vi "array percentage.vi"(8 "path":path=path "D:/Data/20200212_test", 9 "Array":dbl[](array[numeric]), 10 "Judgement value":dbl format="%#_13g") -> ()   [LabVIEW 2018]
uses:
  <vilib>/Utility/file.llb/Read From Spreadsheet File (DBL).vi
panel:
  out "read in array":dbl[](array[numeric])
  # "output the index and element of an array that smaller or equal that judgement value"
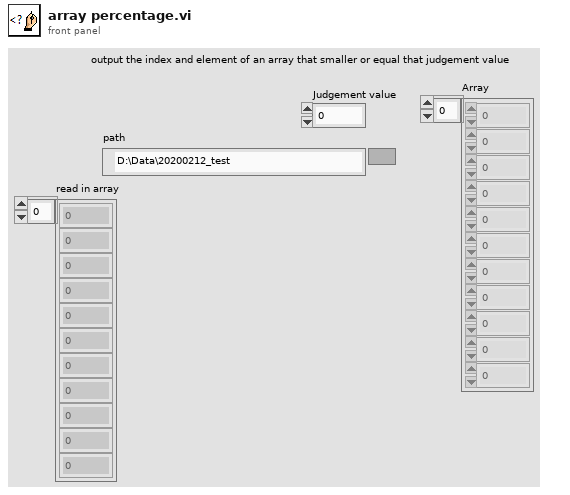
[diagram p1: front panel]
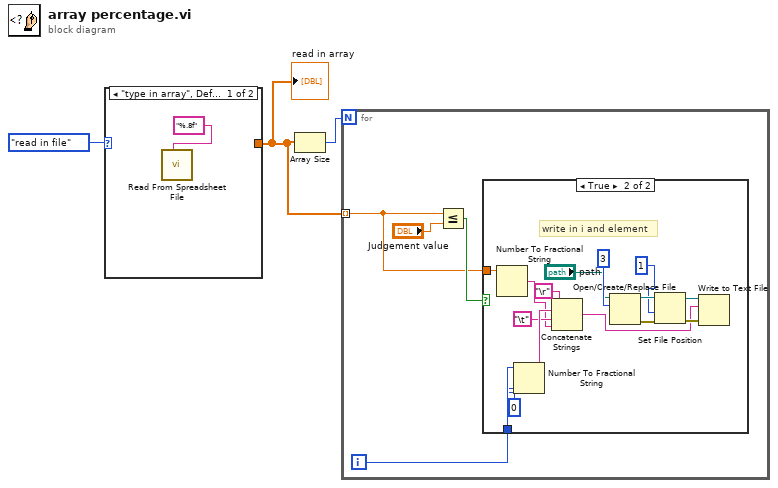
[diagram p0: block diagram]
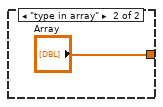
[diagram p2: hidden frame]
diagram:
  n1 = case shown="\"type in array\", Default" enum16{"read in file", "type in array"}."read in file" {
    tunnel: [_ "Array"] -> w2
    frame "type in array", Default {
      n2 = call-poly <vilib>:"Read From Spreadsheet File.vi"("format (%.3f)"="%.8f") -> ()  [unwired: 6 in, 5 out]
    }
    frame "type in array" {
    }
  }
  "read in array" <- w2
  n3 = Array Size(array=w2) -> (size(s)=w3:i32)
  n4 = for {
    N: w3 -> [_]
    tunnel: w2 -> [w6] mode=indexing
    i -> [w7]
    n5 = Less Or Equal?(x=w6, y="Judgement value") -> (x <= y?=w8:bool)
    n6 = case shown="True" w8 {
      tunnel: w7 -> [_ w24]
      tunnel: w6 -> [_ w21]
      frame False {
      }
      frame True {
        # "write in i and element"
        n7 = Number To Fractional String(number=w21) -> (F-format string=w20:string)  [unwired: 3 in]
        n8 = Number To Fractional String(number=w24, precision (6)=0) -> (F-format string=w23:string)  [unwired: 2 in]
        n9 = Concatenate Strings("\r", w23, "\t", w20) -> (w12:string)
        n10 = Open/Create/Replace File(file path (use dialog)="path", operation (0:open)=3) -> (refnum out=w17:refnum<file>, error out=w18:errorcluster)  [unwired: 4 in, 1 out]
        n11 = Set File Position(refnum=w17, from (0:start)=1, error in=w18) -> (refnum out=w14:refnum<file>, error out=w13:errorcluster)  [unwired: 1 in]
        n12 = Write to Text File(file (use dialog)=w14, text=w12, error in=w13) -> ()  [unwired: 1 in, 3 out]
      }
    }
  }
